vi "IncludeProjectLibrary_WhitelistContainsFile.vi"(9 "file":path) -> (0 "error out":errorcluster)   [LabVIEW 2017, in "WhitelistTest.lvlib"]
uses:
  WhitelistTest.lvlib
  Whitelist/Whitelist.lvclass
  Assertion/Assertion.lvlib
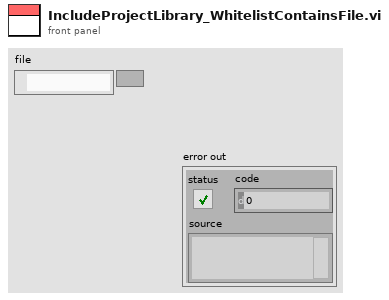
[diagram p1: front panel]
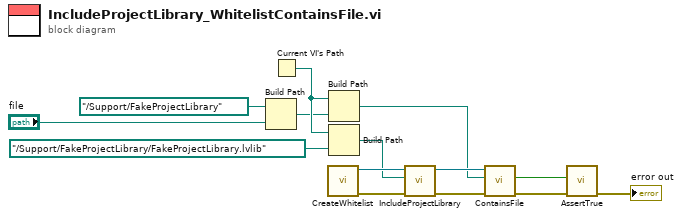
[diagram p0: block diagram]
diagram:
  n1 = Build Path(base path=path "../Support/FakeProjectLibrary", name or relative path="file") -> (appended path=w2:path)
  n2 = Current VI's Path() -> (path=w6:path)
  n3 = call "CreateWhitelist.vi"() -> ("error out"=w13:errorcluster, "Whitelist out"=w14:refnum<class "Whitelist.lvclass">)  [unwired: 10 in]
  n4 = Build Path(base path=w6, name or relative path=w2) -> (appended path=w5:path)
  n5 = Build Path(base path=w6, name or relative path=path "../Support/FakeProjectLibrary/FakeProjectLibrary.lvlib" ("relative_library_path")) -> (appended path=w7:path)
  n6 = call "IncludeProjectLibrary.vi"("error in (no error)"=w13, "Path"=w7, "Whitelist in"=w14) -> ("error out"=w11:errorcluster, "Whitelist out"=w12:refnum<class "Whitelist.lvclass">)  [unwired: 7 in]
  n7 = call "ContainsFile.vi"("error in (no error)"=w11, "Path"=w5, "Whitelist in"=w12) -> ("error out"=w10:errorcluster, "Is Whitelisted?"=w9:bool)  [unwired: 6 in, 1 out]
  n8 = call "AssertTrue.vi"("error in (no error)"=w10, "Condition"=w9) -> ("error out"=→"error out":errorcluster)  [unwired: 9 in]
